vi "Apply filter.vi"(10 "Filter":string, 11 "Item names":string[](array[string])) -> (3 "Filtered Item Names":string[](array[string]))   [LabVIEW 2015, in "TDMS datalogger editor node.lvclass"]
uses:
  TDMS datalogger editor node.lvclass
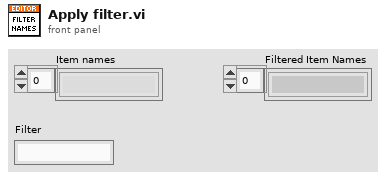
[diagram p1: front panel]
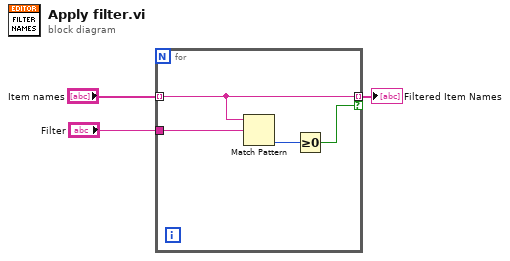
[diagram p0: block diagram]
diagram:
  n1 = for {
    tunnel: "Filter" -> [w7]
    tunnel: [w5] -> w2 mode=indexing if=w6
    tunnel: "Item names" -> [w5] mode=indexing
    n2 = Match Pattern(string=w5, regular expression=w7) -> (offset past match=w4:i32)  [unwired: 1 in, 3 out]
    n3 = Greater Or Equal To 0?(x=w4) -> (x >= 0?=w6:bool)
  }
  "Filtered Item Names" <- w2
